vi "Light_Flashing_1s.vi"(3 "Boolean 3":bool, 4 "Boolean":bool, 5 "Numeric 2":i32) -> (1 "Boolean 2":bool, 2 "Numeric":i32)   [LabVIEW 2016, in "DNP3_Master_Station_MGCC.lvlib"]
uses:
  DNP3_Master_Station_MGCC.lvlib
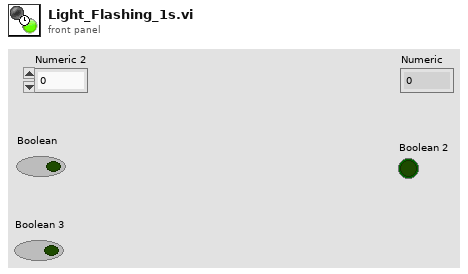
[diagram p1: front panel]
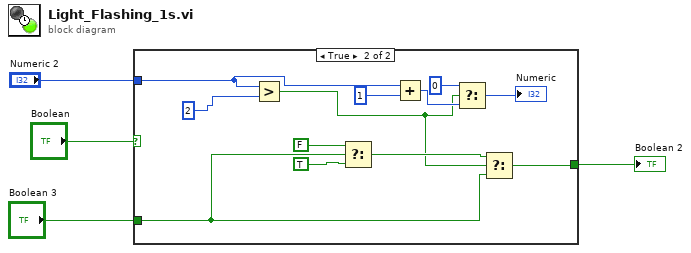
[diagram p0: block diagram]
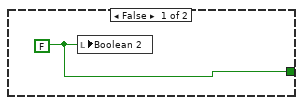
[diagram p2: hidden frame]
diagram:
  n1 = case shown="True" "Boolean" {
    tunnel: [w5 w14] -> w2
    tunnel: "Numeric 2" -> [_ w10]
    tunnel: "Boolean 3" -> [_ w12]
    frame False {
      w5 = FALSE
      n2 = local write "Boolean 2"(w5) -> ()
    }
    frame True {
      n3 = Greater?(x=w10, y=2) -> (0:w7:bool)
      n4 = Select(t=FALSE, s=w12, f=TRUE) -> (s? t:f=w13:bool)
      n5 = Add(x=w10, y=1) -> (x+y=w8:i32)
      n6 = Select(t=0, s=w7, f=w8) -> (s? t:f=→"Numeric":i32)
      n7 = Select(t=w13, s=w7, f=w12) -> (s? t:f=w14:bool)
    }
  }
  "Boolean 2" <- w2
